vi "GetMasterInfo.vi"(4 "数据in":string) -> (0 "主站信息":T1 {"时间戳" format="%016x"; "帧号" format="%04x"; "主站IP" format="%08x"}, 1 "cyclicInfo":i32)   [LabVIEW 2018]
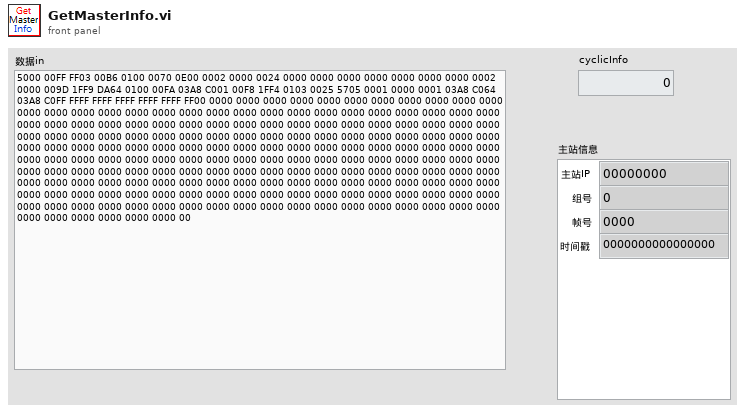
[diagram p1: front panel]
types:
  T1 = cluster{"主站IP":u32, "组号":u8, "帧号":u16, "时间戳":u64}
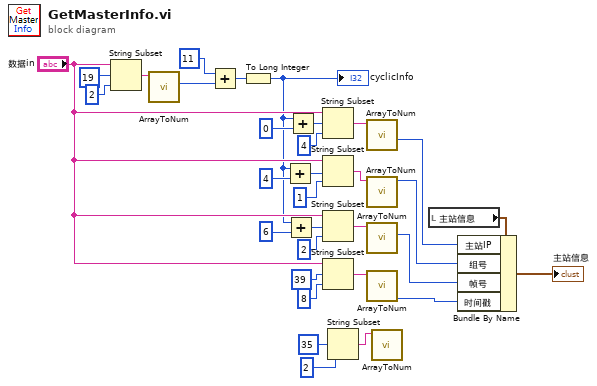
[diagram p0: block diagram]
diagram:
  n1 = String Subset(string="数据in", offset (0)=19 ("长度（剩余）"), length (rest)=2 ("偏移量(0)")) -> (substring=w30:string)
  n2 = call "ArrayToNum.vi"("输入字符串"=w30) -> ("2B"=w29:u16)  [unwired: 3 in, 3 out]
  n3 = Add(x=u16 11, y=w29) -> (x+y=w9:u16)
  n4 = To Long Integer(number=w9) -> (32bit integer=w4:i32)
  "cyclicInfo" <- w4
  n5 = Add(x=w4, y=4 ("索引")) -> (x+y=w8:i32)
  n6 = Add(x=w4, y=6 ("索引")) -> (x+y=w6:i32)
  n7 = Add(x=w4, y=0 ("索引")) -> (x+y=w11:i32)
  n8 = String Subset(string="数据in", offset (0)=w11, length (rest)=4 ("长度")) -> (substring=w27:string)
  n9 = String Subset(string="数据in", offset (0)=w8, length (rest)=1 ("长度")) -> (substring=w26:string)
  n10 = String Subset(string="数据in", offset (0)=w6, length (rest)=2 ("长度")) -> (substring=w25:string)
  n11 = String Subset(string="数据in", offset (0)=39 ("索引"), length (rest)=8 ("长度")) -> (substring=w24:string)
  n12 = String Subset(offset (0)=35 ("偏移量(0)"), length (rest)=2 ("长度（剩余）")) -> (substring=w1:string)  [unwired: 1 in]
  n13 = call "ArrayToNum.vi"("输入字符串"=w27) -> ("4B"=w22:u32)  [unwired: 3 in, 3 out]
  n14 = call "ArrayToNum.vi"("输入字符串"=w26) -> ("1B"=w21:u8)  [unwired: 3 in, 3 out]
  n15 = call "ArrayToNum.vi"("输入字符串"=w25) -> ("2B"=w20:u16)  [unwired: 3 in, 3 out]
  n16 = call "ArrayToNum.vi"("输入字符串"=w24) -> ("8B"=w19:u64)  [unwired: 3 in, 3 out]
  n17 = call "ArrayToNum.vi"("输入字符串"=w1) -> ()  [unwired: 3 in, 4 out]
  n18 = local read "主站信息"() -> (w23:T1)
  n19 = Bundle By Name(cluster=w23, "主站IP"=w22, "组号"=w21, "帧号"=w20, "时间戳"=w19) -> (→"主站信息":T1)
